vi "Set Up Dialog - pH.vi"() -> ()   [LabVIEW 2012]
panel:
  in  "Done":bool
  # "iWorx - pH - Set Up"
  # "Calibration Instructions"
  # "1. Connect the IX-MYDAQ Sensor Adaptor to the NI myDAQ.\n\n2. Connect the PHN-100 pH sensor to the IX-MYDAQ.\n\n3. Connect the NI myDAQ to your computer using a USB cable.\n\n4. Take the boot off of the pH electrode and immerse in a 7.00pH buffer for 30 minutes.\n\n5. After 30 minutes is complete Click set for SP1.\n\n6. Rinse off the electrode and immerse it in a 10.0pH buffer. The 30 minute wait does not need to be repeated here. Click set for SP2."
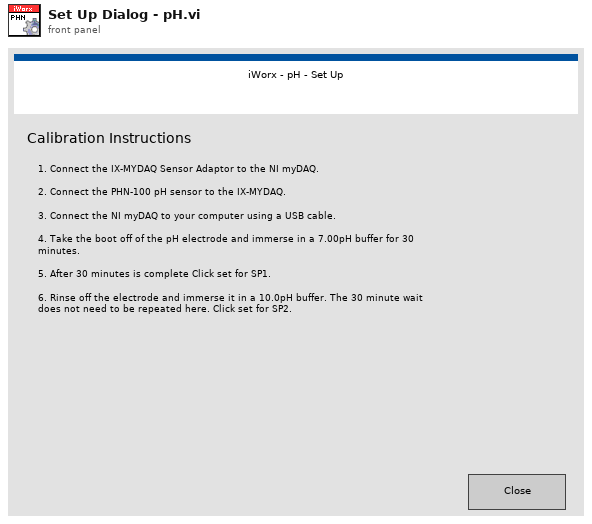
[diagram p1: front panel]
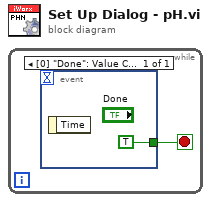
[diagram p0: block diagram]
diagram:
  n1 = while {
    stop <- w1 stop-if-true
    n2 = event shown="[0] \"Done\": Value Change;  Panel Close" {
      selector: _ -> [_]
      dyn-events: _ -> [_]
      timeout: _ -> [_]
      tunnel: [TRUE] -> w1
      event "Done": Value Change; Panel Close {
        n3 = event-data() -> ()  [unwired: 1 in, 1 out]
      }
    }
  }
